vi "get one frame - subvi.vi"(8 "error in":errorcluster, 9 "Image Height":i32, 10 "Image Width":i32, 11 "Image In":T1) -> (0 "error out":errorcluster, 3 "Image Out":T1)   [LabVIEW 2014]
uses:
  <vilib>/vision/Image Controls.llb/IMAQ Image.ctl
  lib/Andorlib/atmcd32d.lvlib
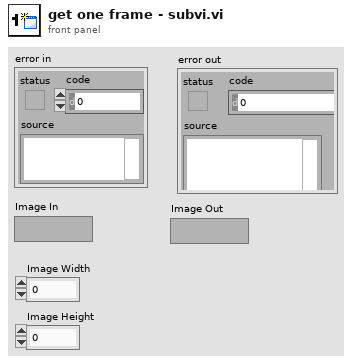
[diagram p1: front panel]
types:
  T1 = typedef "IMAQ Image.ctl" = refnum<image>
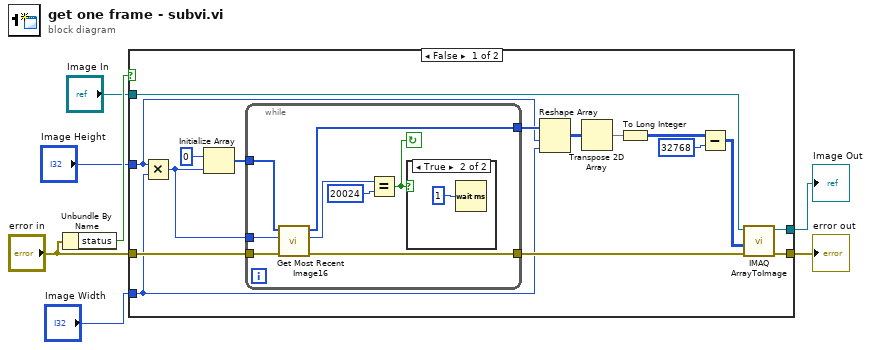
[diagram p0: block diagram]
diagram:
  n1 = Unbundle By Name("error in") -> ("status"=w7:bool)
  n2 = case shown="False" w7 {
    tunnel: "error in" -> [w19 w34]
    tunnel: [w23 w34] -> w2
    tunnel: "Image Height" -> [w14 _]
    tunnel: "Image Width" -> [w13 _]
    tunnel: "Image In" -> [w12 w33]
    tunnel: [w22 w33] -> w1
    frame False {
      n3 = Multiply(x=w14, y=w13) -> (x*y=w16:i32)
      n4 = Initialize Array(u16 0, w16) -> (w17:u16[])
      n5 = while {
        tunnel: [w31] -> w20
        tunnel: w19 -> [w27]
        tunnel: w17 -> [w26]
        tunnel: w16 -> [w25]
        tunnel: [w24] -> w15
        stop <- w28 continue-if-true
        n6 = call "Get Most Recent Image16.vi"("error in (no error)"=w27, "size"=w25, "Array 2"=w26) -> ("error out"=w31:errorcluster, "function return"=w29:u32, "Array"=w24:u16[])  [unwired: 6 in]
        n7 = Equal?(x=w29, y=20024) -> (x = y?=w28:bool)
        n8 = case shown="True" w28 {
          frame False {
          }
          frame True {
            n9 = Wait (ms)(milliseconds to wait=u32 1) -> ()  [unwired: 1 out]
          }
        }
      }
      n10 = Reshape Array(w15, w14, w13) -> (w21:u16[][])
      n11 = Transpose 2D Array(2D array=w21) -> (transposed array=w11:u16[][])
      n12 = To Long Integer(number=w11) -> (32bit integer=w10:i32[][])
      n13 = Subtract(x=w10, y=32768) -> (x-y=w9:i32[][])
      n14 = call "IMAQ ArrayToImage"("error in (no error)"=w20, "Image Pixels (I16)"=w9, "Image"=w12) -> ("error out"=w23:errorcluster, "Image Out"=w22:T1)  [unwired: 3 in, 4 out]
    }
    frame True {
    }
  }
  "error out" <- w2
  "Image Out" <- w1
